vi "getFiducial.vi"(8 "error in (no error)":errorcluster) -> (0 "error out":errorcluster, 1 "coords":sgl, 2 "numFiducials":i32)   [LabVIEW 2011, in "gVision.lvlib"]
uses:
  gVision.lvlib
panel:
  in  "interactive":i32
  in  "colorGroups":i32
  in  "arMax":sgl
  in  "arMin":sgl
  in  "sizeMax":sgl
  in  "sizeMin":sgl
  in  "dilateSize":i32
  in  "shrinkFactor":sgl
  in  "imgHeight":i32
  in  "imgWidth":i32
  in  "imgLineWidth":i32
  in  "img":string
  in  "return type":i32
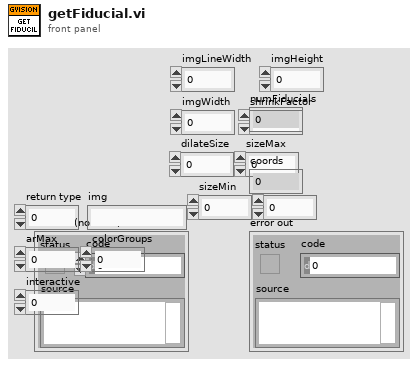
[diagram p1: front panel]
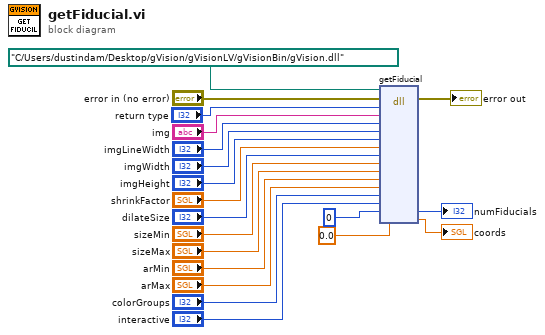
[diagram p0: block diagram]
diagram:
  n1 = dll-call lib="C:/Users/dustindam/Desktop/gVision/gVisionLV/gVisionBin/gVision.dll" fn="getFiducial"(path in=path "C:/Users/dustindam/Desktop/gVision/gVisionLV/gVisionBin/gVision.dll", error in="error in (no error)", "return type"="return type", "img"="img", "imgLineWidth"="imgLineWidth", "imgWidth"="imgWidth", "imgHeight"="imgHeight", "shrinkFactor"="shrinkFactor", "dilateSize"="dilateSize", "sizeMin"="sizeMin", "sizeMax"="sizeMax", "arMin"="arMin", "arMax"="arMax", "colorGroups"="colorGroups", "interactive"="interactive", "numFiducials"=0, "coords"=sgl 0.0) -> (error out=→"error out":errorcluster, "numFiducials"=→"numFiducials":i32, "coords"=→"coords":sgl)  [unwired: 13 in, 1 out]
